vi "Generate Timed Ramp.vi"(4 "Log":bool, 5 "Point #":i32, 6 "Time (Hr:Min:Sec)":dbl=60.0 format="%<%H:%M:%S>t", 7 "Stop":dbl=10.0, 8 "Start":dbl) -> (0 "Stop":bool, 1 "Valid":bool, 2 "Time Remaining":dbl=60.0 format="%<%H:%M:%S>t", 3 "Output":dbl format="%.3f")   [LabVIEW 2020]
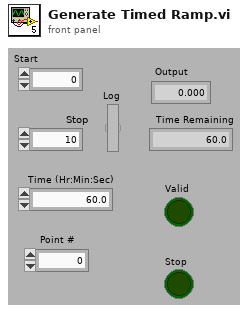
[diagram p1: front panel]
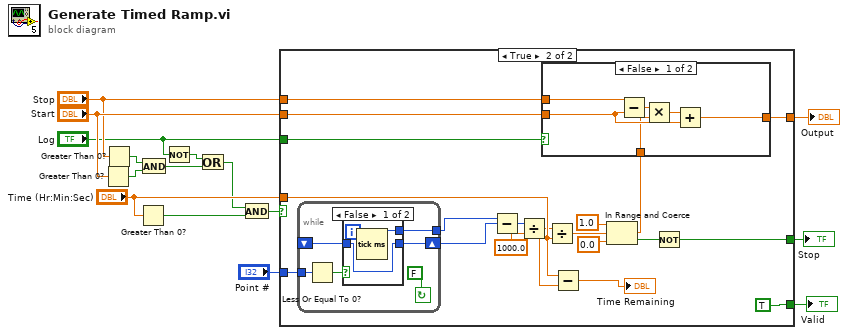
[diagram p0: block diagram]
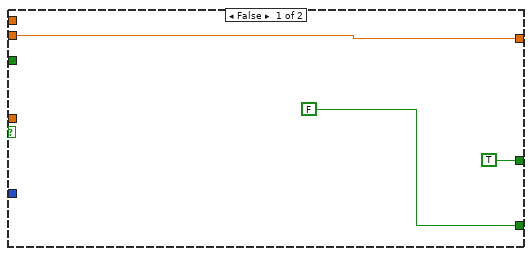
[diagram p2: hidden frame]
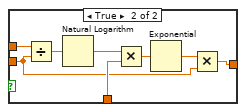
[diagram p3: hidden frame]
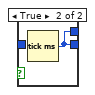
[diagram p4: hidden frame]
diagram:
  n1 = Greater Than 0?(x="Start") -> (x > 0?=w6:bool)
  n2 = Greater Than 0?(x="Stop") -> (x > 0?=w7:bool)
  n3 = Greater Than 0?(x="Time (Hr:Min:Sec)") -> (x > 0?=w13:bool)
  n4 = And(x=w7, y=w6) -> (x .and. y?=w5:bool)
  n5 = Not(x="Log") -> (.not. x?=w3:bool)
  n6 = Or(x=w3, y=w5) -> (x .or. y?=w4:bool)
  n7 = And(x=w4, y=w13) -> (x .and. y?=w10:bool)
  n8 = case shown="True" w10 {
    tunnel: "Time (Hr:Min:Sec)" -> [_ w21]
    tunnel: "Stop" -> [_ w34]
    tunnel: "Start" -> [w16 w33]
    tunnel: "Point #" -> [_ w32]
    tunnel: [w16 w31] -> w12
    tunnel: [FALSE ("Valid") TRUE ("Valid")] -> w11
    tunnel: "Log" -> [_ w25]
    tunnel: [TRUE w23] -> w1
    frame False {
    }
    frame True {
      n9 = while {
        shift-left: _ -> [w55]
        shift-right: [w56] -> w37
        tunnel: w32 -> [w53]
        tunnel: [w52] -> w22
        stop <- FALSE continue-if-true
        n10 = Less Or Equal To 0?(x=w53) -> (x <= 0?=w57:bool)
        n11 = case shown="False" w57 {
          tunnel: [w58 w60] -> w56
          tunnel: w55 -> [w58 _]
          tunnel: [w59 w60] -> w52
          frame False {
            n12 = Tick Count (ms)() -> (millisecond timer value=w59:u32)
          }
          frame True {
            n13 = Tick Count (ms)() -> (millisecond timer value=w60:u32)
          }
        }
      }
      n14 = Subtract(x=w22, y=w37) -> (x-y=w36:u32)
      n15 = Divide(x=w36, y=1000.0) -> (x/y=w20:dbl)
      n16 = Divide(x=w20, y=w21) -> (x/y=w29:dbl)
      n17 = Subtract(x=w21, y=w20) -> (x-y=→"Time Remaining":dbl)
      n18 = In Range and Coerce(upper limit=1.0, x=w29, lower limit=0.0) -> (coerced(x)=w26:dbl, In Range?=w24:bool)
      n19 = case shown="False" w25 {
        tunnel: w34 -> [w41 w48]
        tunnel: w33 -> [w40 w45]
        tunnel: [w39 w44] -> w31
        tunnel: w26 -> [w38 w47]
        frame False {
          n20 = Subtract(x=w41, y=w40) -> (x-y=w43:dbl)
          n21 = Multiply(x=w43, y=w38) -> (x*y=w42:dbl)
          n22 = Add(x=w42, y=w40) -> (x+y=w39:dbl)
        }
        frame True {
          n23 = Divide(x=w48, y=w45) -> (x/y=w51:dbl)
          n24 = Natural Logarithm(1:w51) -> (0:w46:dbl)
          n25 = Multiply(x=w46, y=w47) -> (x*y=w50:dbl)
          n26 = Exponential(1:w50) -> (0:w49:dbl)
          n27 = Multiply(x=w49, y=w45) -> (x*y=w44:dbl)
        }
      }
      n28 = Not(x=w24) -> (.not. x?=w23:bool)
    }
  }
  "Output" <- w12
  "Valid" <- w11
  "Stop" <- w1
